vi "Set INTENSITY.vi"(8 "error in (no error)":errorcluster caption="entrée d'erreur (pas d'erreur)", 10 "INTENSITY":u32, 11 "Class Instrument LED_Analyser en entrée":refnum<class "Class Instrument LED_Analyser.lvclass">) -> (0 "error out":errorcluster caption="sortie d'erreur", 3 "Class Instrument LED_Analyser en sortie":refnum<class "Class Instrument LED_Analyser.lvclass">)   [LabVIEW 2020, in "Library Instrument & Equipement.lvlib" / "Library Instruments.lvlib" / "Class Instrument LED_Analyser.lvclass"]
uses:
  Class Instrument LED_Analyser.lvclass
  Class Instrument LED_Analyser.lvclass/Class Instrument LED_Analyser.ctl
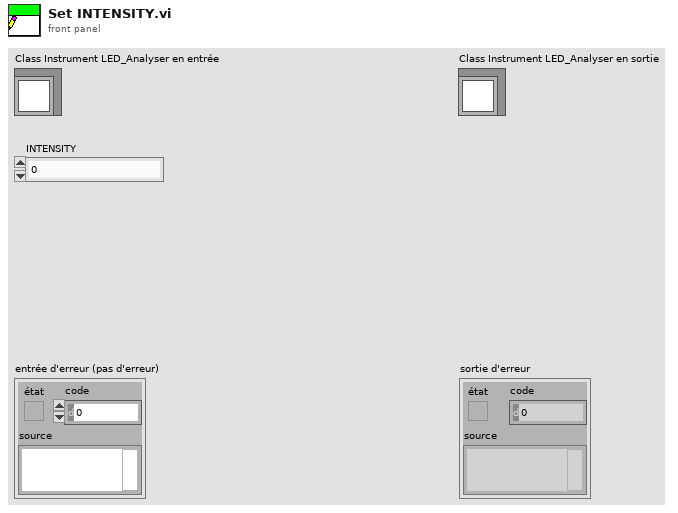
[diagram p1: front panel]
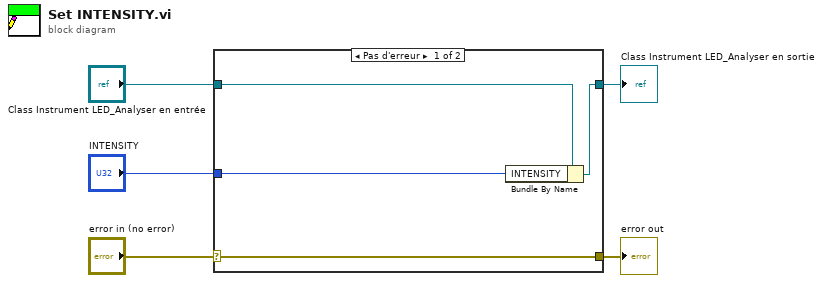
[diagram p0: block diagram]
diagram:
  n1 = case shown="Pas d'erreur" "error in (no error)" {
    selector: "error in (no error)" -> [w9 w10]
    tunnel: [w9 w10] -> w4
    tunnel: [w7 w11] -> w2
    tunnel: "Class Instrument LED_Analyser en entrée" -> [w8 w11]
    tunnel: "INTENSITY" -> [w6 _]
    frame No Error {
      n2 = Bundle By Name(cluster=w8, "INTENSITY"=w6) -> (w7:refnum<class "Class Instrument LED_Analyser.lvclass">)
    }
    frame Error {
    }
  }
  "error out" <- w4
  "Class Instrument LED_Analyser en sortie" <- w2
